vi "tm_gettimestamp.vi"(8 "error in (no error)":errorcluster, 10 "Frame Index":i32=-1, 11 "File Handle in":u32) -> (0 "error out":errorcluster, 2 "Timestamp":dbl, 3 "File Handle out":u32)   [LabVIEW 2012]
uses:
  tmcamcon.dll
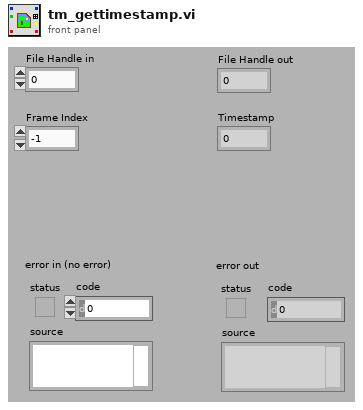
[diagram p1: front panel]
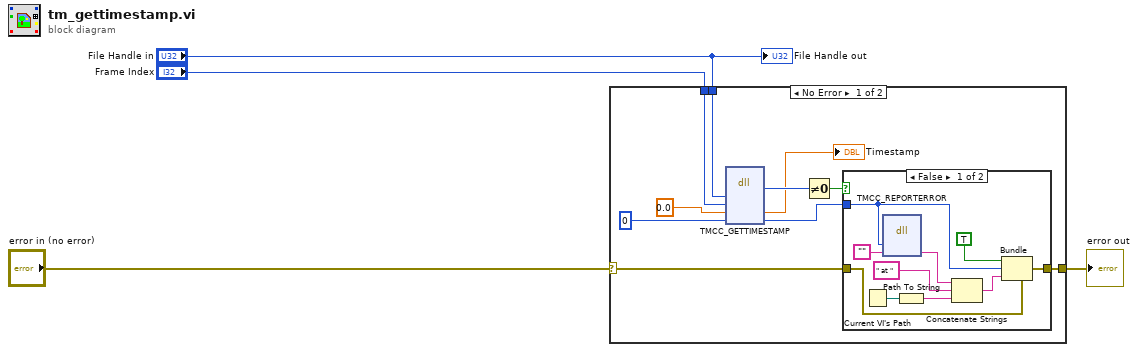
[diagram p0: block diagram]
diagram:
  n1 = case shown="No Error" "error in (no error)" {
    selector: "error in (no error)" -> [w11 w26]
    tunnel: [w10 w26] -> w3
    tunnel: "File Handle in" -> [w9 _]
    tunnel: "Frame Index" -> [w8 _]
    frame No Error {
      n2 = dll-call lib="tmcamcon.dll" fn="TMCC_GETTIMESTAMP"("index"=w9, "frame"=w8, "timestamp"=0.0 ("Erval"), "Erval"=0) -> ("return type"=w14:u32, "timestamp"=→"Timestamp":dbl, "Erval"=w12:i32)  [unwired: 5 in, 2 out]
      n3 = Not Equal To 0?(x=w14) -> (x != 0?=w13:bool)
      n4 = case shown="False" w13 {
        tunnel: w11 -> [w24 w25]
        tunnel: [w23 w25] -> w10
        tunnel: w12 -> [w17 _]
        frame False {
          n5 = Current VI's Path() -> (path=w22:path)
          n6 = dll-call lib="tmcamcon.dll" fn="TMCC_REPORTERROR"("error"=w17, "buf"="") -> ("buf"=w16:string)  [unwired: 5 in, 2 out]
          n7 = Path To String(path=w22) -> (string=w18:string)
          n8 = Concatenate Strings(w16, " at ", w18) -> (w21:string)
          n9 = Bundle(cluster=w24, "status"=TRUE, "code"=w17, "source"=w21) -> (w23:errorcluster)
        }
        frame True {
        }
      }
    }
    frame Error {
    }
  }
  "error out" <- w3
  "File Handle out" <- "File Handle in"
